vi "LVClass_ClosedLoopSecurityActivation_Dtor.vi"(0 "ClosedLoopSecurityActivation in":refnum<class "ClosedLoopSecurityActivation.lvclass">, 11 "error in (no error)":errorcluster) -> (4 "ClosedLoopSecurityActivation out":refnum<class "ClosedLoopSecurityActivation.lvclass">, 15 "error out":errorcluster)   [LabVIEW 2020, in "ClosedLoopSecurityActivation.lvclass"]
doc: "Destruction.\n\n<B>security_activationIn</B> : Pointer to Closed Loop security activation object.\n<B>security_activationOut</B> : Pointer to Closed Loop security activation object."
uses:
  ClosedLoopSecurityActivation.lvclass
  ClosedLoopSecurityActivation.lvclass/ClosedLoopSecurityActivation.ctl
  Controls/Handle creation.ctl
  Controls/ClassID.ctl
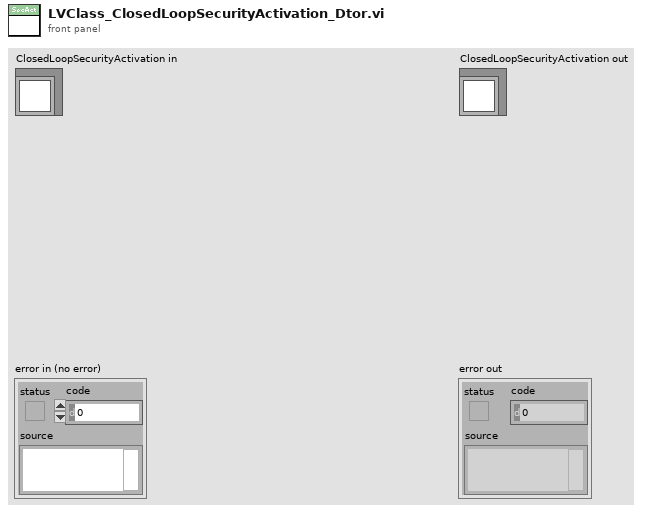
[diagram p1: front panel]
types:
  T1 = typedef "ClassID.ctl" = i64
  T2 = typedef "Handle creation.ctl" = enum16{"By ctor", "By write function"}
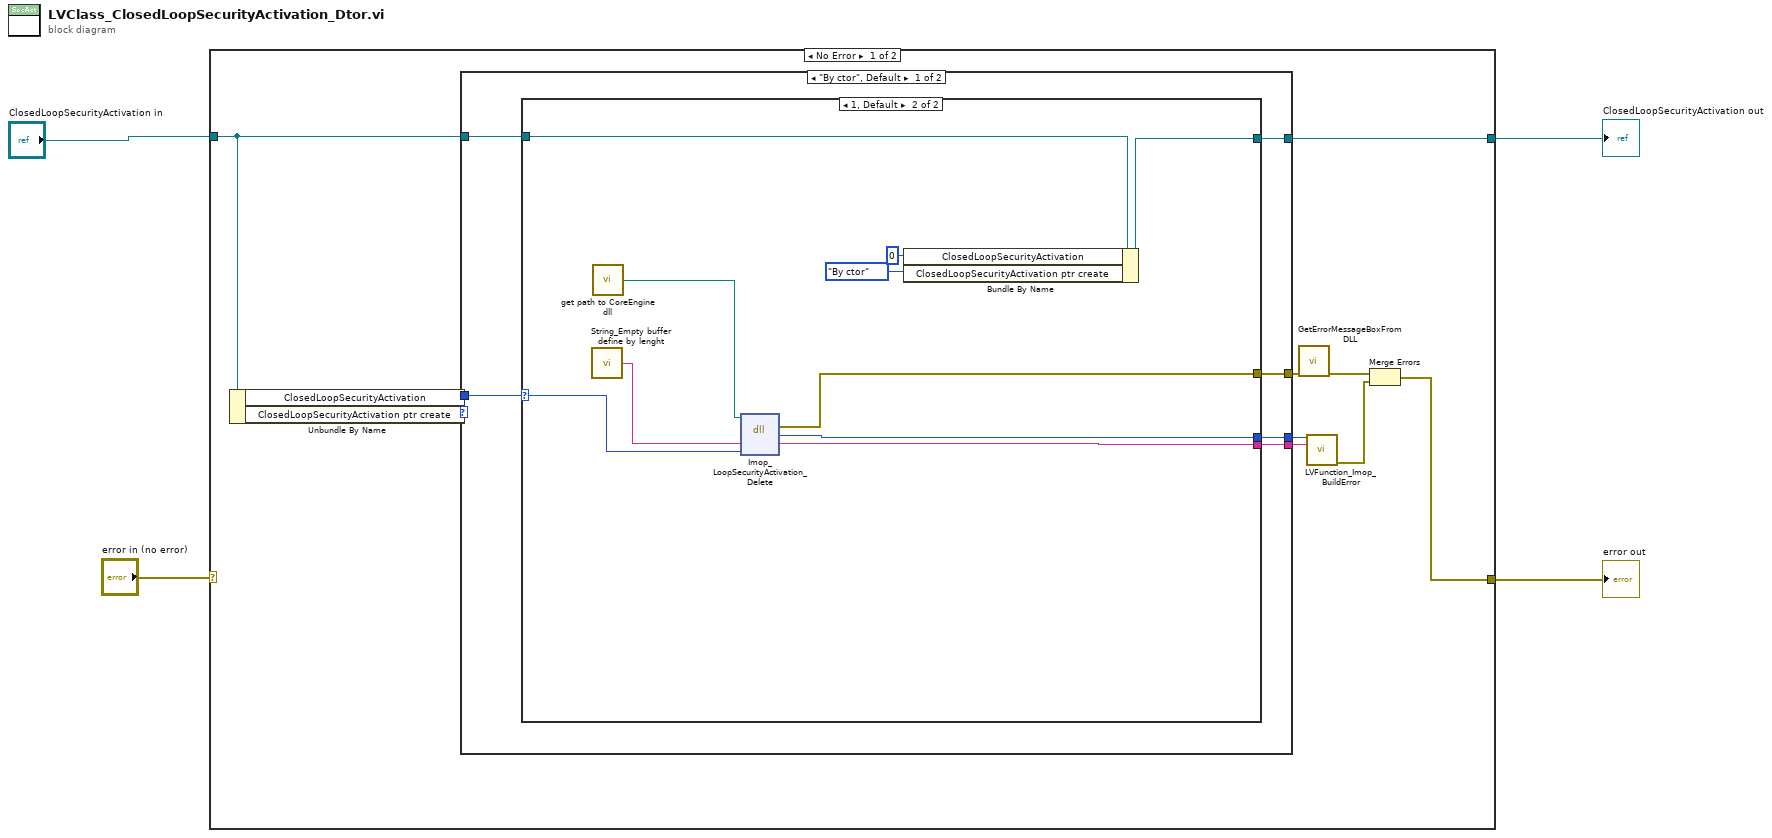
[diagram p0: block diagram]
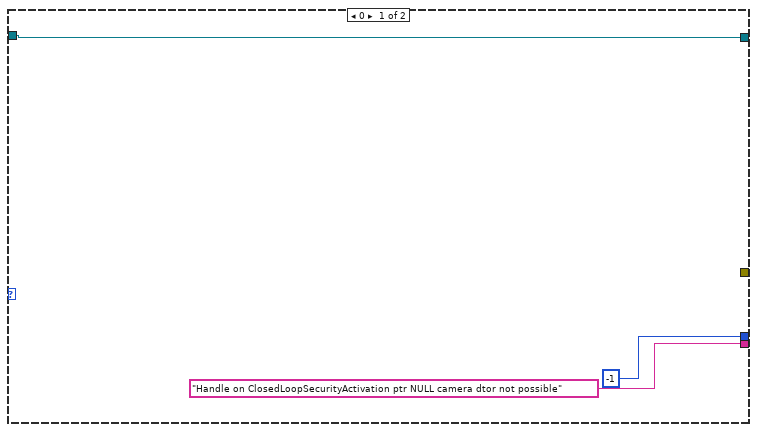
[diagram p2: hidden frame]
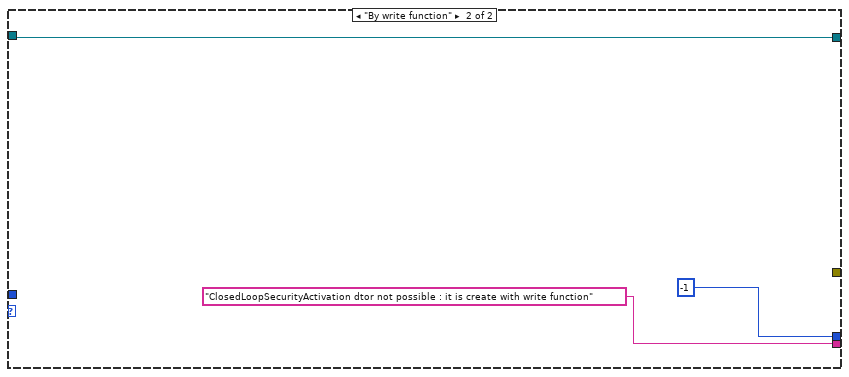
[diagram p3: hidden frame]
diagram:
  n1 = case shown="No Error" "error in (no error)" {
    selector: "error in (no error)" -> [_ w38]
    tunnel: [w8 w38] -> w3
    tunnel: [w9 w37] -> w1
    tunnel: "ClosedLoopSecurityActivation in" -> [w7 w37]
    frame No Error {
      n2 = Unbundle By Name(w7) -> ("ClosedLoopSecurityActivation"=w6:T1, "ClosedLoopSecurityActivation ptr create"=w5:T2)
      n3 = case shown="\"By ctor\", Default" w5 {
        tunnel: [w20 "ClosedLoopSecurityActivation dtor not possible : it is create with write function" ("message")] -> w14
        tunnel: [w19 -1] -> w13
        tunnel: [w18 _] -> w12
        tunnel: w7 -> [w17 w36]
        tunnel: [w16 w36] -> w9
        tunnel: w6 -> [w15 _]
        frame "By ctor", Default {
          n4 = case shown="1, Default" w15 {
            selector: w15 -> [_ w25]
            tunnel: ["Handle on ClosedLoopSecurityActivation ptr NULL camera dtor not possible" ("message") w32] -> w20
            tunnel: [-1 w31] -> w19
            tunnel: [_ w30] -> w18
            tunnel: w17 -> [w23 w27]
            tunnel: [w23 w26] -> w16
            frame 0 {
            }
            frame 1, Default {
              n5 = call "String_Empty buffer define by lenght.vi"() -> ("Empty buffer"=w33:string)  [unwired: 1 in]
              n6 = call "get path to CoreEngine dll.vi"() -> ("path to wavekit library"=w28:path)  [unwired: 14 in, 1 out]
              n7 = dll-call lib="D:/soft/HASO_v3/SVN_trunk/ImOpCoreEngine4_LV2011/DLLs/c_interface_vc100.dll" fn="Imop_LoopSecurityActivation_Delete"(path in=w28, "message"=w33, "security_activation"=w25) -> (error out=w30:errorcluster, "return type"=w31:i32, "message"=w32:string)  [unwired: 3 in, 1 out]
              n8 = Bundle By Name(cluster=w27, "ClosedLoopSecurityActivation"=T1 0, "ClosedLoopSecurityActivation ptr create"=Handle_creation."By ctor" ("Pupil ptr create")) -> (w26:refnum<class "ClosedLoopSecurityActivation.lvclass">)
            }
          }
        }
        frame "By write function" {
        }
      }
      n9 = call "GetErrorMessageBoxFromDLL.vi"("error IN"=w12) -> ("error OUT"=w11:errorcluster)  [unwired: 10 in]
      n10 = call "LVFunction_Imop_BuildError.vi"("code"=w13, "String to Prepend to source (\"\")"=w14) -> ("error out"=w10:errorcluster)  [unwired: 13 in]
      n11 = Merge Errors(w11, w10) -> (w8:errorcluster)
    }
    frame Error {
    }
  }
  "error out" <- w3
  "ClosedLoopSecurityActivation out" <- w1
